vi "FTW-Request-Receive.vi"(0 "Uninitialized Request":refnum<class "FTW-Request.lvclass">, 11 "error in":errorcluster) -> (4 "Initialized Request":refnum<class "FTW-Request.lvclass">, 6 "Request Header":string, 15 "error out":errorcluster)   [LabVIEW 2013, in "FTW-Actor.lvlib" / "FTW-Request.lvclass"]
uses:
  FTW-Request.lvclass
  FTW-Request.lvclass/FTW-Request.ctl
  Core/src/JSON/FTW-JSON.lvclass
panel:
  # "Inputs"
  # "Outputs"
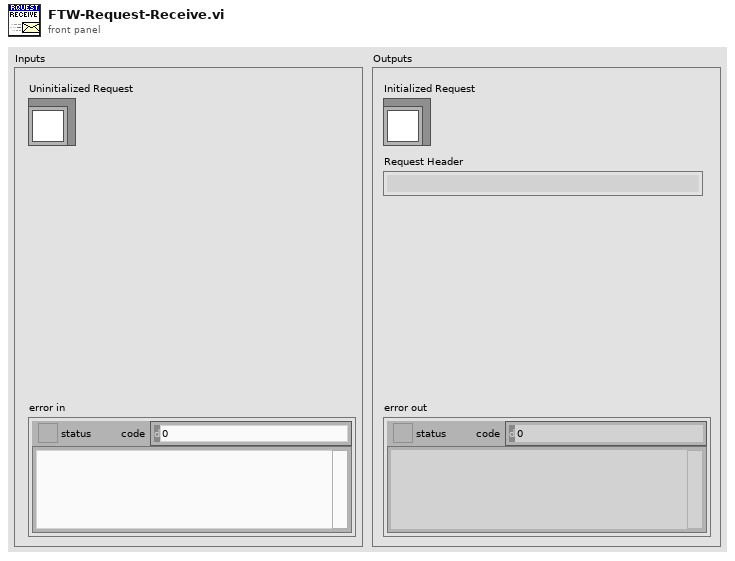
[diagram p1: front panel]
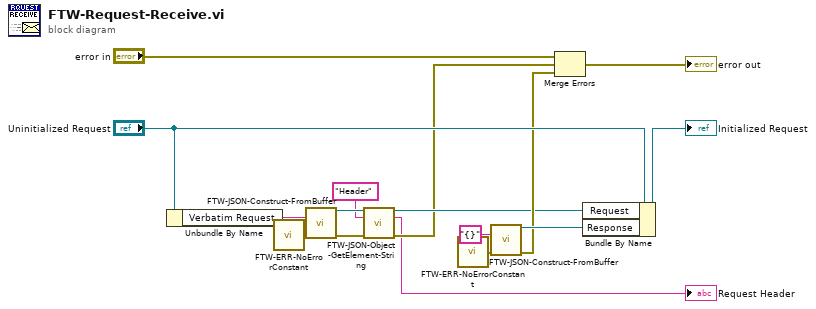
[diagram p0: block diagram]
diagram:
  n1 = Unbundle By Name("Uninitialized Request") -> ("Verbatim Request"=w14:string)
  n2 = call "FTW-ERR-NoErrorConstant.vi"() -> ("no error"=w12:errorcluster)
  n3 = call "FTW-JSON-Construct-FromBuffer.vi"("JSON String (UTF-8)"=w14, "error in"=w12) -> ("JSON Object"=w6:refnum<class "FTW-JSON.lvclass">, "error out"=w4:errorcluster)  [unwired: 12 in]
  n4 = call "FTW-JSON-Object-GetElement-String.vi"("JSON Object"=w6, "Key"="Header", "error in"=w4) -> ("JSON Object out"=w5:refnum<class "FTW-JSON.lvclass">, "Value"=→"Request Header":string, "error out"=w3:errorcluster)  [unwired: 9 in, 1 out]
  n5 = call "FTW-ERR-NoErrorConstant.vi"() -> ("no error"=w11:errorcluster)
  n6 = call "FTW-JSON-Construct-FromBuffer.vi"("JSON String (UTF-8)"="{}", "error in"=w11) -> ("JSON Object"=w13:refnum<class "FTW-JSON.lvclass">, "error out"=w7:errorcluster)  [unwired: 12 in]
  n7 = Merge Errors("error in", w3, w7) -> (→"error out":errorcluster)
  n8 = Bundle By Name(cluster="Uninitialized Request", "Request"=w5, "Response"=w13) -> (→"Initialized Request":refnum<class "FTW-Request.lvclass">)
